vi "Stop.vi"(8 "error in (no error)":errorcluster, 9 "Channel Data (DBLs Only)":T1, 10 "Real-Time System Data":T2, 11 "Configuration Data":T3) -> (0 "error out":errorcluster)   [LabVIEW 2014, in "RM interrupt timing Custom Device.lvlib"]
uses:
  RM interrupt timing Custom Device.lvlib
  Configuration Data.ctl
  Real-Time System Data.ctl
  Channel Data.ctl
  <instrlib>/GE 5565 PIORC/GE 5565 PIORC.lvlib
panel:
  # "Controls"
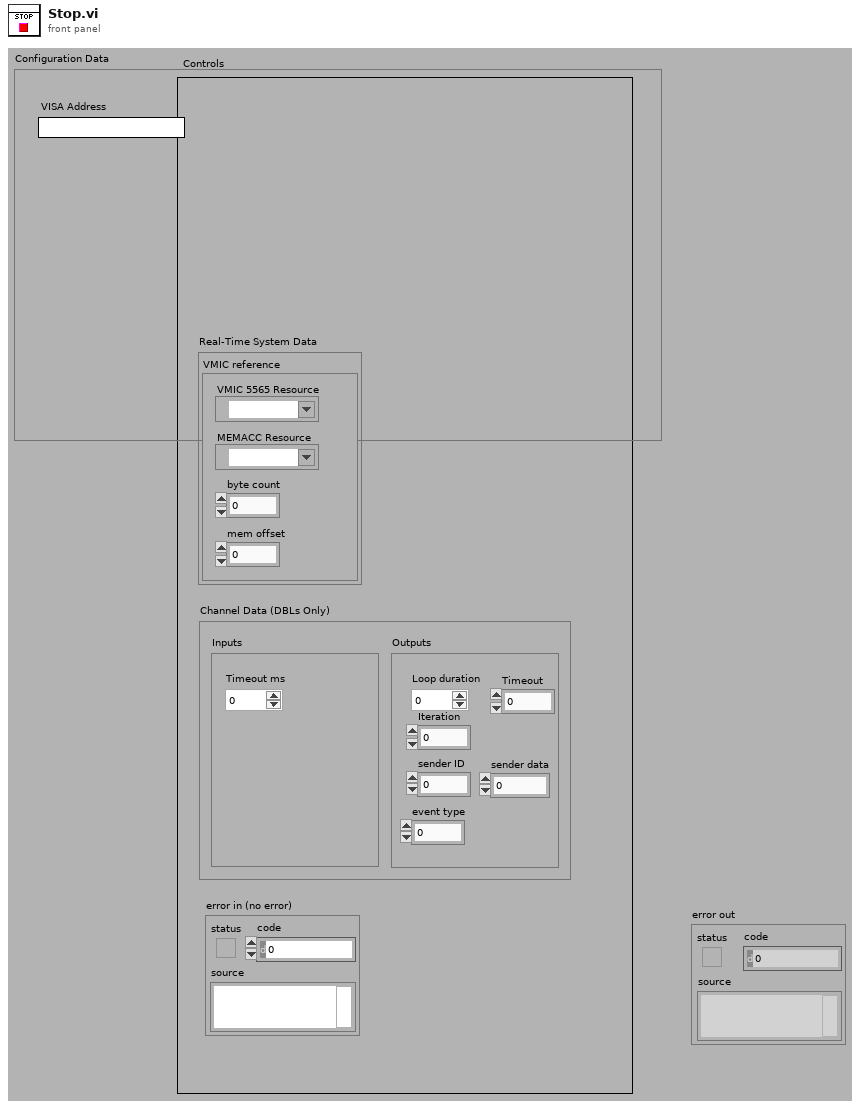
[diagram p1: front panel]
types:
  T1 = typedef "RM interrupt timing Custom Device.lvlib/Channel Data.ctl" = cluster{"Inputs":cluster{"Timeout ms":dbl}, "Outputs":cluster{"Loop duration":dbl, "Iteration":dbl, "Timeout":dbl, "sender data":dbl, "sender ID":dbl, "event type":dbl}}
  T2 = typedef "RM interrupt timing Custom Device.lvlib/Real-Time System Data.ctl" = cluster{"VMIC reference":cluster{"VMIC 5565 Resource":refnum<visa-resource-name>, "MEMACC Resource":refnum<visa-resource-name>, "byte count":u32, "mem offset":u32}}
  T3 = typedef "RM interrupt timing Custom Device.lvlib/Configuration Data.ctl" = cluster{"VISA Address":string}
  T4 = enum16{"link reset interrupt", "network interrupt 1", "network interrupt 2", "network interrupt 3", "network init interrupt", "all"}
  T5 = cluster{"VMIC 5565 Resource":refnum<visa-resource-name>, "MEMACC Resource":refnum<visa-resource-name>, "byte count":u32, "mem offset":u32}
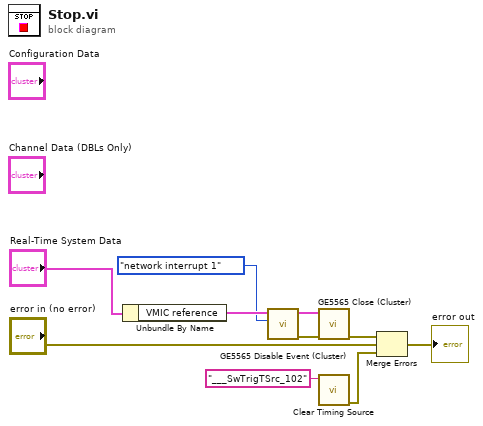
[diagram p0: block diagram]
diagram:
  n1 = Unbundle By Name("Real-Time System Data") -> ("VMIC reference"=w7:T5)
  n2 = call <instrlib>:"GE5565 Disable Event (Cluster).vi"("event type (all)"=T4."network interrupt 1", "VMIC reference in"=w7) -> ("error out"=w10:errorcluster, "VMIC reference out"=w9:T5)  [unwired: 4 in]
  n3 = call <instrlib>:"GE5565 Close (Cluster).vi"("error in (no error)"=w10, "VMIC reference in"=w9) -> ("error out"=w6:errorcluster)  [unwired: 5 in]
  n4 = call <vilib>:"Clear Timing Source.vi"("name"="___SwTrigTSrc_102") -> ("error out"=w1:errorcluster)  [unwired: 9 in, 1 out]
  n5 = Merge Errors(w6, "error in (no error)", w1) -> (→"error out":errorcluster)
